vi "test random.vi"() -> ()   [LabVIEW 2018, in "LV2Julia_core.lvlib"]
uses:
  LV2Julia_core.lvlib
  8ff801c8-b98c-4af1-845c-0726e8db660c.vi
  8ff801c8-b98c-4af1-845c-0726e8db660c.vi/978c6eef-4b37-4e43-87a2-7d168b27b768.vi
panel:
  in  "arr size":u32
  out "Bool out":bool[](array[boolean])
  out "float out":dbl[](array[numeric])
  in  "type in":dbl
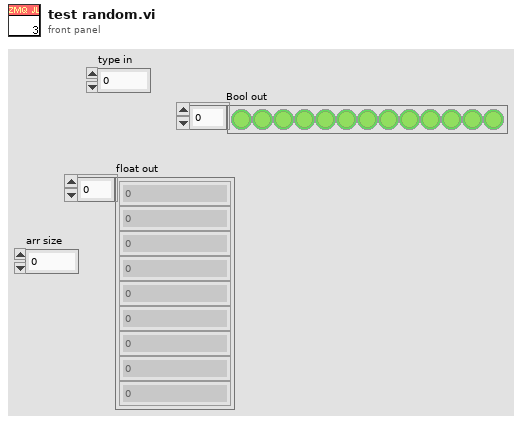
[diagram p1: front panel]
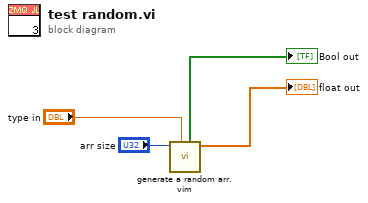
[diagram p0: block diagram]
diagram:
  n1 = call "generate a random arr.vim"("type in"="type in", "arr size"="arr size") -> ("float out"=→"float out":dbl[], "Bool out"=→"Bool out":bool[])  [unwired: 5 in, 3 out]
